vi "vPage_9234x2_CHx8(by71).vi"() -> ()   [LabVIEW 2018]
uses:
  <vilib>/Utility/sysdir.llb/System Directory Type.ctl
  <vilib>/express/express analysis/Spectral/Block/exnSpectralBlock spectral measurements peak poly.vi
  <vilib>/express/express analysis/Spectral/Block/exnSpectralBlock spectral measurements peak DDT.vi
  <vilib>/express/express analysis/Spectral/XNode/ExpressSpectralMeasurementsBlockNode.xnode
panel:
  in  "Show":bool
  out "DAQ Stoped":bool
  out "C1":i32
  out "C2":i32
  in  "SW \n(C1-C2)":bool[](array[boolean])=[TRUE, TRUE, TRUE, TRUE, TRUE, TRUE, TRUE, TRUE]
  in  "Filter(Hz)\nLow-Cut":dbl=10.0
  in  "Sample \nto Read":i32=6400
  in  "Sample\nRate":dbl=6400.0
  in  "資料夾\n註記>":string
  in  "Enable Saving":bool
  in  "Stop":bool
  out "C1-Save":bool
  out "C1-Trigger":bool
  in  "Show_FFT":bool
  out "C1-All":dynamicdata(graph)
  out "C2-All":dynamicdata(graph)
  out "C1-0":dynamicdata(graph)
  out "C2-0":dynamicdata(graph)
  out "C1-1":dynamicdata(graph)
  out "C2-1":dynamicdata(graph)
  out "C1-2":dynamicdata(graph)
  out "C2-2":dynamicdata(graph)
  out "C1-3":dynamicdata(graph)
  out "C2-3":dynamicdata(graph)
  # "使用前請先確認 \nDAQ 擷取卡設定"
  # "本頁畫面顯示為 觸發後訊號"
  # "FFT Filter by useing High-pass with Lower Cut-Off (Hz)"
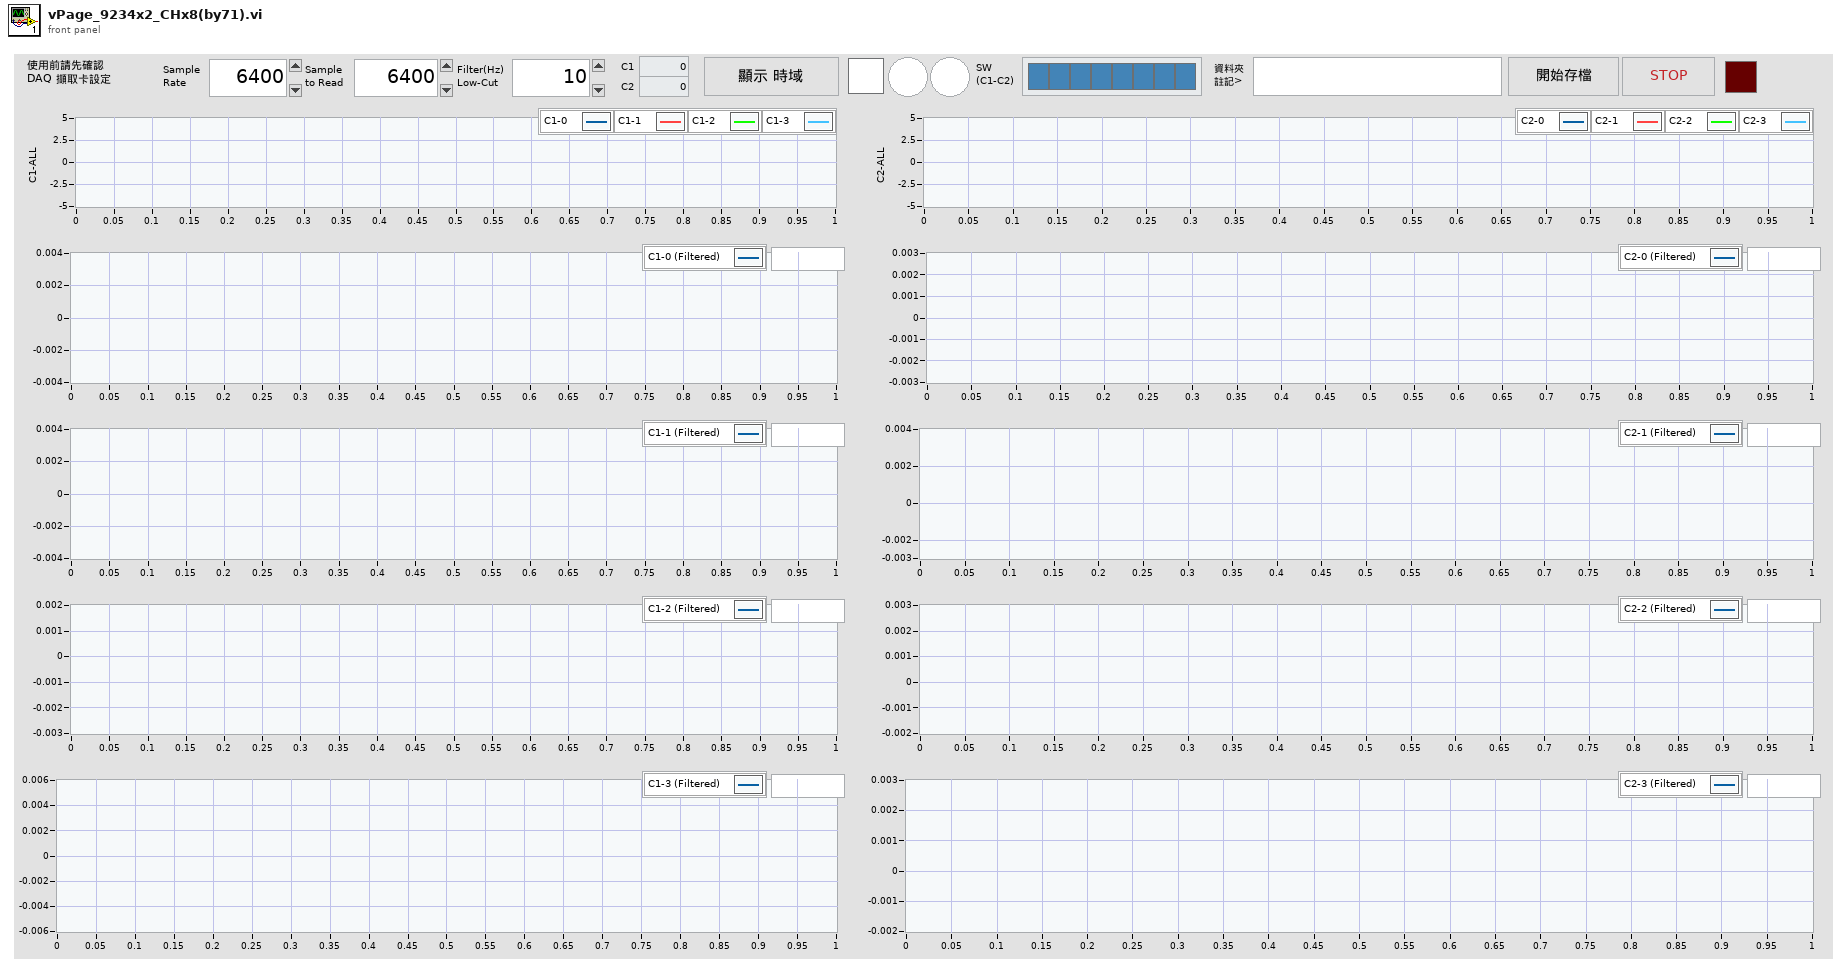
[diagram p1: front panel]
types:
  T1 = enum8{"Enabled", "Disabled", "Disabled and Grayed Out"}
  T2 = typedef "System Directory Type.ctl" = i32
  T3 = cluster{"task out":refnum<k21>, "data":dynamicdata}
  T4 = cluster{"averaging mode":u16, "weighting mode":u16, "number of averages":u32}
  T5 = cluster{"dB On (F)":bool, "unwrap phase (F)":bool, "convert to degree (F)":bool}
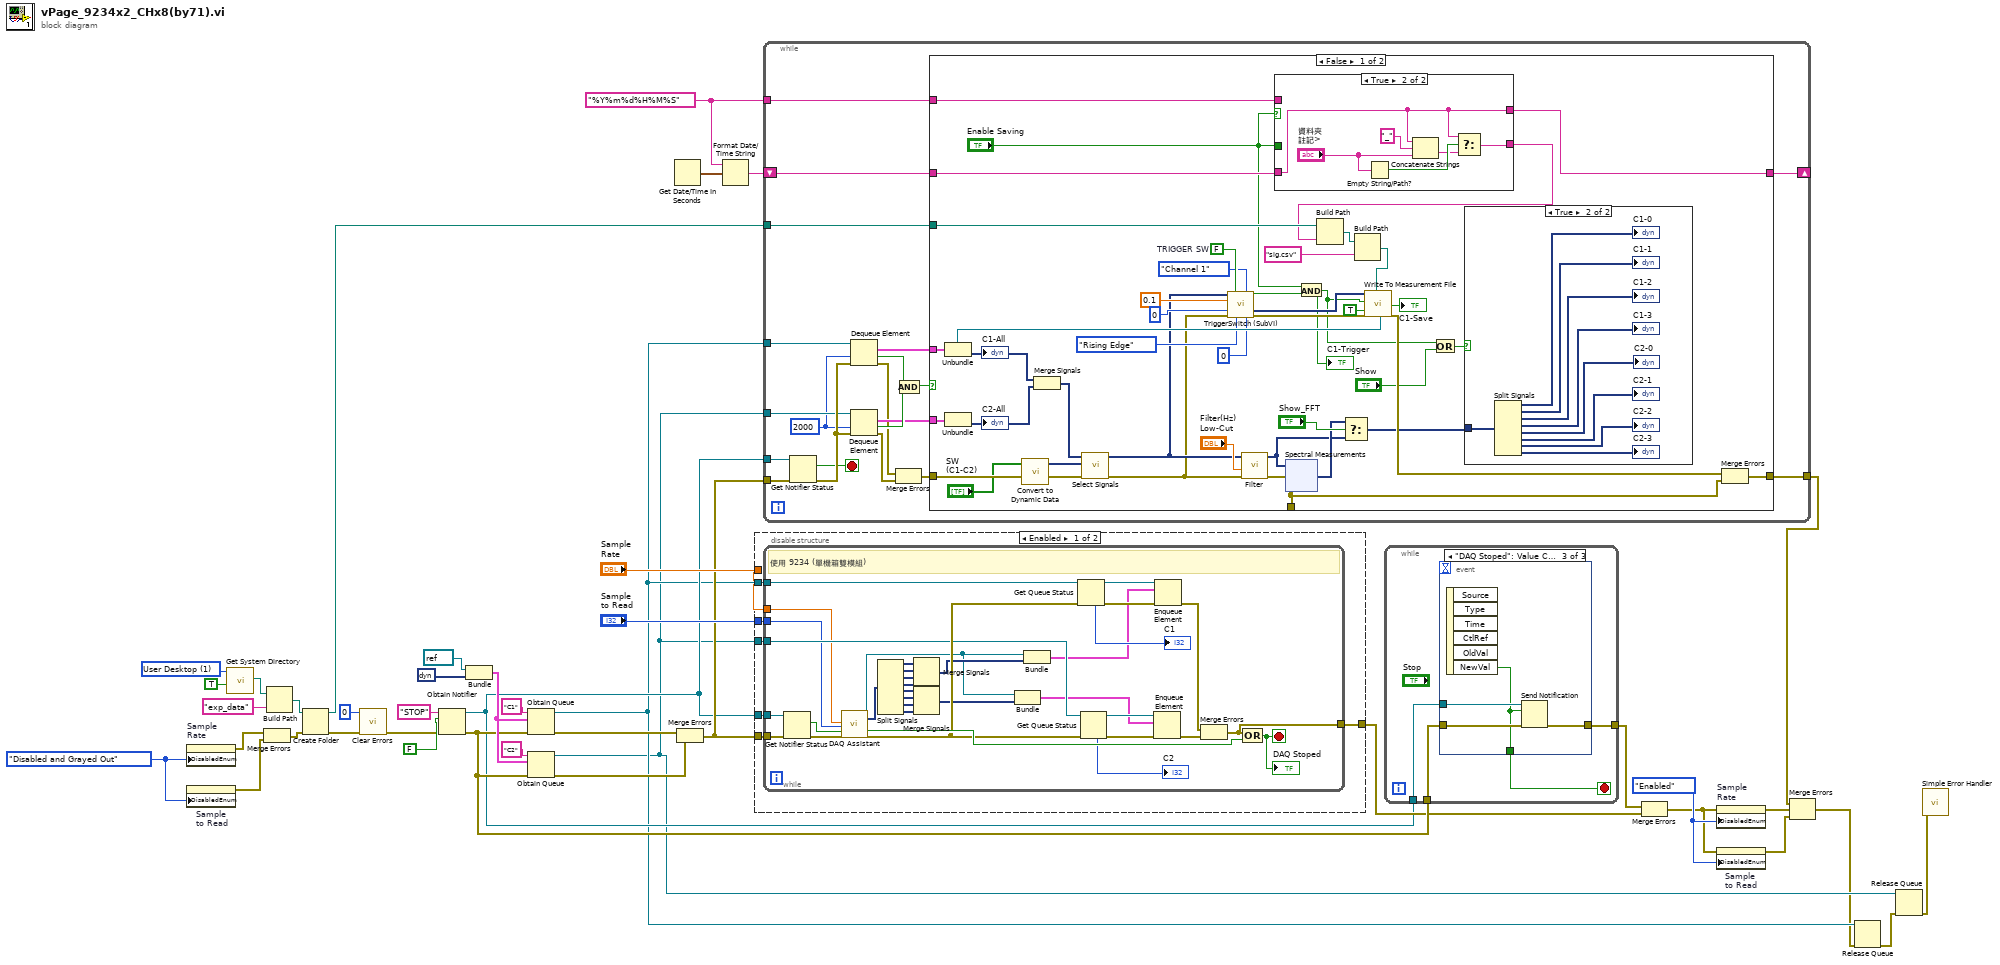
[diagram p0: block diagram]
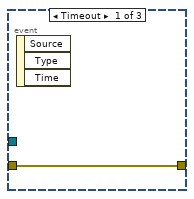
[diagram p2: hidden frame]
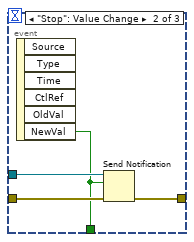
[diagram p3: hidden frame]
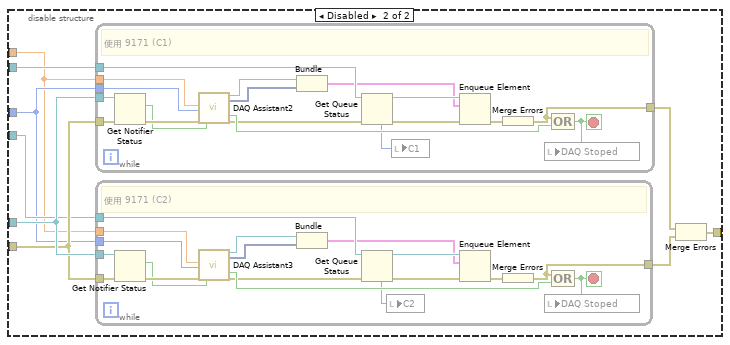
[diagram p4: hidden frame]
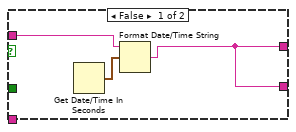
[diagram p6: hidden frame]
diagram:
  w10 = T1."Enabled" ("Disabled")
  w14 = T1."Disabled and Grayed Out" ("Disabled")
  w15 = "%Y%m%d%H%M%S" ("time format string (%c)")
  w25 = T2 1 items=["User Home"=0, "User Desktop"=1, "User Documents"=2, "User Application Data"=3, "User Preferences"=4, "User Temporary"=5, "Public Documents"=6, "Public Application Data"=7, "Public Preferences"=8, "Public Cache"=13, "System Core Libraries"=9, "System Installed Libraries"=10, "Application Files"=11, "Boot Volume Root"=12] ("system directory type")
  n1 = property on="Sample\nRate" class="DigNum (strict)"("DisabledEnum"=w14) -> (error out=w13:errorcluster)  [unwired: 2 in, 1 out]
  n2 = property on="Sample \nto Read" class="DigNum (strict)"("DisabledEnum"=w14) -> (error out=w11:errorcluster)  [unwired: 2 in, 1 out]
  n3 = call <vilib>:"Get System Directory.vi"("create directory if not found? (F)"=TRUE, "system directory type"=w25) -> ("system directory"=w27:path)  [unwired: 9 in]
  n4 = Merge Errors(w13, w11) -> (w12:errorcluster)
  n5 = Build Path(base path=w27, name or relative path="exp_data") -> (appended path=w21:path)
  n6 = Create Folder(path (use dialog)=w21, error in=w12) -> (created path=w20:path, error out=w23:errorcluster)  [unwired: 1 in, 1 out]
  n7 = call <vilib>:"Clear Errors.vi"("error in (no error)"=w23, "specific error code to clear (0: all)"=0) -> ("error out"=w22:errorcluster)  [unwired: 4 in, 1 out]
  n8 = Obtain Notifier(name (unnamed)="STOP", notification data type=FALSE, error in (no error)=w22) -> (notifier out=w16:refnum<notifier>, error out=w19:errorcluster)  [unwired: 1 in, 1 out]
  n9 = Bundle("task out"=refnum<k21> refnum, "data"=dynamicdata []) -> (w32:T3)  [unwired: 1 in]
  n10 = Obtain Queue(name (unnamed)="C1", element data type=w32, error in (no error)=w19) -> (queue out=w5:refnum<queue>, error out=w42:errorcluster)  [unwired: 2 in, 1 out]
  n11 = Obtain Queue(name (unnamed)="C2", element data type=w32, error in (no error)=w19) -> (queue out=w4:refnum<queue>, error out=w41:errorcluster)  [unwired: 2 in, 1 out]
  n12 = Get Date/Time In Seconds() -> (seconds since 1Jan1904=w30:timestamp)
  n13 = Merge Errors(w42, w41) -> (w31:errorcluster)
  n14 = Format Date/Time String(time format string (%c)=w15, seconds (now)=w30) -> (date/time string=w29:string)  [unwired: 1 in]
  n15 = disable-structure shown="Enabled" {
    disable-tunnel: w5 -> [w49 w89]
    disable-tunnel: w4 -> [w48 w90]
    disable-tunnel: w31 -> [w47 w91]
    disable-tunnel: w16 -> [w46 w92]
    disable-tunnel: "Sample \nto Read" -> [w45 w88]
    disable-tunnel: "Sample\nRate" -> [w44 w87]
    disable-tunnel: [w43 w85] -> w17
    frame Enabled {
      n16 = while {
        tunnel: [w74] -> w43
        tunnel: w48 -> [w66]
        tunnel: w49 -> [w65]
        tunnel: w47 -> [w64]
        tunnel: w46 -> [w63]
        tunnel: w45 -> [w56]
        tunnel: w44 -> [w55]
        stop <- w72 stop-if-true
        # "使用 9234 (單機箱雙模組)"
        n17 = Get Notifier Status(notifier=w63, error in (no error)=w64) -> (current notification=w80:bool, error out=w81:errorcluster)  [unwired: 3 out]
        n18 = call "DAQ Assistant"("rate"=w55, "number of samples"=w56, "error in"=w81, "stop (F)"=w80) -> ("task out"=w59:refnum<k21>, "data"=w71:dynamicdata, "stopped"=w79:bool, "error out"=w78:errorcluster)  [unwired: 12 in]
        n19 = Split Signals(w71) -> (w70:dynamicdata, w69:dynamicdata, w68:dynamicdata, w54:dynamicdata, w53:dynamicdata, w52:dynamicdata, w51:dynamicdata, w50:dynamicdata)  [unwired: 8 in]
        n20 = Merge Signals(w70, w69, w68, w54) -> (w60:dynamicdata)
        n21 = Merge Signals(w53, w52, w51, w50) -> (w61:dynamicdata)
        n22 = Bundle("task out"=w59, w61) -> (w58:cluster{"task out":refnum<k21>, dynamicdata})  [unwired: 1 in]
        n23 = Bundle("task out"=w59, w60) -> (w57:cluster{"task out":refnum<k21>, dynamicdata})  [unwired: 1 in]
        n24 = Get Queue Status(queue=w65, error in (no error)=w78) -> (queue out=w62:refnum<queue>, error out=w77:errorcluster, # elements in queue=→"C1":i32)  [unwired: 1 in, 5 out]
        n25 = Get Queue Status(queue=w66, error in (no error)=w78) -> (queue out=w83:refnum<queue>, error out=w82:errorcluster, # elements in queue=→"C2":i32)  [unwired: 1 in, 5 out]
        n26 = Enqueue Element(queue=w83, element=w58, error in (no error)=w82) -> (error out=w76:errorcluster)  [unwired: 1 in, 2 out]
        n27 = Enqueue Element(queue=w62, element=w57, error in (no error)=w77) -> (error out=w75:errorcluster)  [unwired: 1 in, 2 out]
        n28 = Merge Errors(w75, w76) -> (w74:errorcluster)
        n29 = Compound Arithmetic op=OR(w74, w79) -> (w72:bool)
        "DAQ Stoped" <- w72
      }
    }
    frame Disabled {
      n30 = while {
        tunnel: [w121] -> w84
        tunnel: w92 -> [w120]
        tunnel: w91 -> [w119]
        tunnel: w89 -> [w118]
        tunnel: w88 -> [w115]
        tunnel: w87 -> [w114]
        stop <- w116 stop-if-true
        # "使用 9171 (C1)"
        n31 = Get Notifier Status(notifier=w120, error in (no error)=w119) -> (current notification=w125:bool, error out=w126:errorcluster)  [unwired: 3 out]
        n32 = call "DAQ Assistant2"("rate"=w114, "number of samples"=w115, "error in"=w126, "stop (F)"=w125) -> ("task out"=w113:refnum<k21>, "data"=w112:dynamicdata, "stopped"=w124:bool, "error out"=w123:errorcluster)  [unwired: 12 in]
        n33 = Bundle("task out"=w113, "data"=w112) -> (w111:T3)  [unwired: 1 in]
        n34 = Get Queue Status(queue=w118, error in (no error)=w123) -> (queue out=w128:refnum<queue>, error out=w127:errorcluster, # elements in queue=w117:i32)  [unwired: 1 in, 5 out]
        n35 = local write "C1"(w117) -> ()
        n36 = Enqueue Element(queue=w128, element=w111, error in (no error)=w127) -> (error out=w122:errorcluster)  [unwired: 1 in, 2 out]
        n37 = Merge Errors(w122) -> (w121:errorcluster)
        n38 = Compound Arithmetic op=OR(w121, w124) -> (w116:bool)
        n39 = local write "DAQ Stoped"(w116) -> ()
      }
      n40 = while {
        tunnel: [w103] -> w86
        tunnel: w92 -> [w102]
        tunnel: w91 -> [w101]
        tunnel: w90 -> [w100]
        tunnel: w88 -> [w97]
        tunnel: w87 -> [w96]
        stop <- w98 stop-if-true
        # "使用 9171 (C2)"
        n41 = Get Notifier Status(notifier=w102, error in (no error)=w101) -> (current notification=w107:bool, error out=w108:errorcluster)  [unwired: 3 out]
        n42 = call "DAQ Assistant3"("rate"=w96, "number of samples"=w97, "error in"=w108, "stop (F)"=w107) -> ("task out"=w94:refnum<k21>, "data"=w95:dynamicdata, "stopped"=w106:bool, "error out"=w105:errorcluster)  [unwired: 12 in]
        n43 = Bundle("task out"=w94, "data"=w95) -> (w93:T3)  [unwired: 1 in]
        n44 = Get Queue Status(queue=w100, error in (no error)=w105) -> (queue out=w110:refnum<queue>, error out=w109:errorcluster, # elements in queue=w99:i32)  [unwired: 1 in, 5 out]
        n45 = local write "C2"(w99) -> ()
        n46 = Enqueue Element(queue=w110, element=w93, error in (no error)=w109) -> (error out=w104:errorcluster)  [unwired: 1 in, 2 out]
        n47 = Merge Errors(w104) -> (w103:errorcluster)
        n48 = Compound Arithmetic op=OR(w103, w106) -> (w98:bool)
        n49 = local write "DAQ Stoped"(w98) -> ()
      }
      n50 = Merge Errors(w84, w86) -> (w85:errorcluster)
    }
  }
  n51 = while {
    tunnel: w31 -> [w148]
    tunnel: w16 -> [w146]
    tunnel: w5 -> [w145]
    tunnel: w4 -> [w144]
    shift-right: [w133] -> _
    shift-left: w29 -> [w134]
    tunnel: w20 -> [w132]
    tunnel: [w131] -> w2
    tunnel: w15 -> [w129]
    stop <- w130 stop-if-true
    w143 = 2000 ("timeout in ms (-1)")
    n52 = Get Notifier Status(notifier=w146, error in (no error)=w148) -> (current notification=w130:bool, error out=w147:errorcluster)  [unwired: 3 out]
    n53 = Dequeue Element(queue=w145, timeout in ms (-1)=w143, error in (no error)=w147) -> (element=w139:T3, timed out?=w141:bool, error out=w137:errorcluster)  [unwired: 1 out]
    n54 = Dequeue Element(queue=w144, timeout in ms (-1)=w143, error in (no error)=w147) -> (element=w138:T3, timed out?=w142:bool, error out=w136:errorcluster)  [unwired: 1 out]
    n55 = Merge Errors(w137, w136) -> (w135:errorcluster)
    n56 = And(x=w141, y=w142) -> (x .and. y?=w140:bool)
    n57 = case shown="False" w140 {
      tunnel: w139 -> [w189 _]
      tunnel: w138 -> [w188 _]
      tunnel: w135 -> [w185 w220]
      tunnel: [w163 _] -> _
      tunnel: w134 -> [w171 w221]
      tunnel: [w170 w221] -> w133
      tunnel: w132 -> [w169 _]
      tunnel: [w162 w220] -> w131
      tunnel: w129 -> [w152 _]
      frame False {
        w182 = FALSE  # TRIGGER SW
        n58 = Unbundle(w189) -> ("task out"=w183:refnum<k21>, "data"=w187:dynamicdata)
        "C1-All" <- w187
        n59 = Unbundle(w188) -> ("data"=w186:dynamicdata)  [unwired: 1 out]
        "C2-All" <- w186
        n60 = call "Convert to Dynamic Data"("Array"="SW \n(C1-C2)") -> ("Dynamic Data Type"=w157:dynamicdata)  [unwired: 3 in]
        n61 = Merge Signals(w187, w186) -> (w184:dynamicdata)
        n62 = call "Select Signals"("error in (no error)"=w185, "Selector Input"=w157, "Signals"=w184) -> ("error out"=w173:errorcluster, "Signal Out"=w176:dynamicdata)  [unwired: 7 in]
        n63 = call "TriggerSwitch (SubVI).vi"("data"=w176, "TRIGGER SW"=w182, "Trigger Axis"=enum32{"Channel 1", "Channel 2", "Channel 3"}."Channel 1", "Trigger Level"=0.1, "Samples to Read"=0, "error in (no error)"=w173, "Trigger Slope"=enum16{"Falling Edge", "Rising Edge"}."Rising Edge", "Pre Samples"=0) -> ("Data Available"=w174:bool, "Section"=w175:dynamicdata, "error out"=w172:errorcluster)  [unwired: 5 in]
        n64 = call "Filter"("error in (no error)"=w173, "Lower Cut-Off"="Filter(Hz)\nLow-Cut", "Signal"=w176) -> ("error out"=w191:errorcluster, "Filtered Signal"=w159:dynamicdata)  [unwired: 7 in]
        n65 = case shown="True" "Enable Saving" {
          tunnel: [w201 w204] -> w170
          tunnel: "Enable Saving" -> [_ _]
          tunnel: w171 -> [_ w204]
          tunnel: [w201 w206] -> w153
          tunnel: w152 -> [w202 _]
          frame False {
            n66 = Get Date/Time In Seconds() -> (seconds since 1Jan1904=w203:timestamp)
            n67 = Format Date/Time String(time format string (%c)=w202, seconds (now)=w203) -> (date/time string=w201:string)  [unwired: 1 in]
          }
          frame True {
            n68 = Empty String/Path?(string/path="資料夾\n註記>") -> (empty?=w208:bool)
            n69 = Concatenate Strings(w204, "_" ("string"), "資料夾\n註記>") -> (w207:string)
            n70 = Select(t=w204, s=w208, f=w207) -> (s? t:f=w206:string)
          }
        }
        n71 = xnode ("Spectral Measurements")("Signals"=w159, "error in (no error)"=w191) -> ("FFT - (Peak)"=w160:dynamicdata, "error out"=w163:errorcluster)  [unwired: 1 out]
        n72 = And(x="Enable Saving", y=w174) -> (x .and. y?=w151:bool)
        "C1-Trigger" <- w151
        n73 = Build Path(base path=w169, name or relative path=w153) -> (appended path=w168:path)
        n74 = Select(t=w160, s="Show_FFT", f=w159) -> (s? t:f=w156:dynamicdata)
        n75 = Build Path(base path=w168, name or relative path="sig.csv") -> (appended path=w166:path)
        n76 = call "Write To Measurement File"("Signals"=w175, "Enable"=w151, "new_file"=TRUE, "error in (no error)"=w172, "Filename"=w166, "DAQmx Task"=w183) -> ("Saving Data"=→"C1-Save":bool, "error out"=w164:errorcluster)  [unwired: 11 in, 1 out]
        n77 = Or(x=w151, y="Show") -> (x .or. y?=w150:bool)
        n78 = case shown="True" w150 {
          tunnel: w156 -> [_ w200]
          frame False {
          }
          frame True {
            n79 = Split Signals(w200) -> (→"C1-0":dynamicdata, →"C1-1":dynamicdata, →"C1-2":dynamicdata, →"C1-3":dynamicdata, →"C2-0":dynamicdata, →"C2-1":dynamicdata, →"C2-2":dynamicdata, →"C2-3":dynamicdata)  [unwired: 8 in]
          }
        }
        n80 = Merge Errors(w164, w163) -> (w162:errorcluster)
      }
      frame True {
      }
    }
  }
  n81 = while {
    tunnel: w19 -> [w225]
    tunnel: [w224] -> w18
    tunnel: w16 -> [w223]
    stop <- w222 stop-if-true
    n82 = event shown="[2] \"DAQ Stoped\": Value Change" {
      selector: _ -> [_ _ _]
      dyn-events: _ -> [_ _ _]
      timeout: _ -> [_ _ _]
      tunnel: w225 -> [w226 w230 w234]
      tunnel: [w226 w229 w233] -> w224
      tunnel: w223 -> [_ w228 w232]
      tunnel: [_ w227 w231] -> w222
      event Timeout {
        n83 = event-data() -> ()  [unwired: 1 in, 3 out]
      }
      event "Stop": Value Change {
        n84 = event-data() -> ("NewVal"=w227:bool)  [unwired: 1 in, 5 out]
        n85 = Send Notification(notification=w227, notifier=w228, error in (no error)=w230) -> (error out=w229:errorcluster)  [unwired: 1 out]
      }
      event "DAQ Stoped": Value Change {
        n86 = event-data() -> ("NewVal"=w231:bool)  [unwired: 1 in, 5 out]
        n87 = Send Notification(notification=w231, notifier=w232, error in (no error)=w234) -> (error out=w233:errorcluster)  [unwired: 1 out]
      }
    }
  }
  n88 = Merge Errors(w18, w17) -> (w6:errorcluster)
  n89 = property on="Sample\nRate" class="DigNum (strict)"(error in=w6, "DisabledEnum"=w10) -> (error out=w9:errorcluster)  [unwired: 1 in, 1 out]
  n90 = property on="Sample \nto Read" class="DigNum (strict)"(error in=w6, "DisabledEnum"=w10) -> (error out=w8:errorcluster)  [unwired: 1 in, 1 out]
  n91 = Merge Errors(w2, w9, w8) -> (w1:errorcluster)
  n92 = Release Queue(queue=w5, error in (no error)=w1) -> (error out=w7:errorcluster)  [unwired: 1 in, 2 out]
  n93 = Release Queue(queue=w4, error in (no error)=w7) -> (error out=w3:errorcluster)  [unwired: 1 in, 2 out]
  n94 = call <vilib>:"Simple Error Handler.vi"("error in (no error)"=w3) -> ()  [unwired: 4 in, 5 out]
